vi "To Serial Form.vi"(6 "Serial Version":T1, 10 "Serializer in":refnum<class "Serializer.lvclass">, 11 "CRDS Cell Data in":refnum<class "CRDS Cell Data.lvclass">) -> (0 "error out":errorcluster, 2 "Serializer out":refnum<class "Serializer.lvclass">, 3 "CRDS Cell Data out":refnum<class "CRDS Cell Data.lvclass">)   [LabVIEW 2014, in "CRDS Cell Data.lvclass"]
uses:
  CRDS Cell Data.lvclass
  <vilib>/NI/AQ Character Lineator/Serializer/Serializer.lvclass
  <vilib>/NI/AQ Character Lineator/Serialization Common/Serial Version.ctl
  CRDS Cell Data.lvclass/CRDS Cell Data.ctl
  <vilib>/NI/AQ Character Lineator/Serializable/Insert Single.vi
  <vilib>/NI/AQ Character Lineator/Serializable/Insert Int16 Array.vi
  <vilib>/NI/AQ Character Lineator/Serializable/Insert Single Array.vi
  <vilib>/NI/AQ Character Lineator/Serializer/Insert Single.vi
  <vilib>/NI/AQ Character Lineator/Serializer/Insert Int16 Array.vi
  <vilib>/NI/AQ Character Lineator/Serializer/Insert Single Array.vi
  <vilib>/NI/AQ Character Lineator/Serializer/Read Include Default Values.vi
  Data/Data.lvclass
  <vilib>/NI/AQ Character Lineator/Serializable/Serializable.lvclass
  <vilib>/NI/AQ Character Lineator/Serialization Common/Serialization Common.lvlib
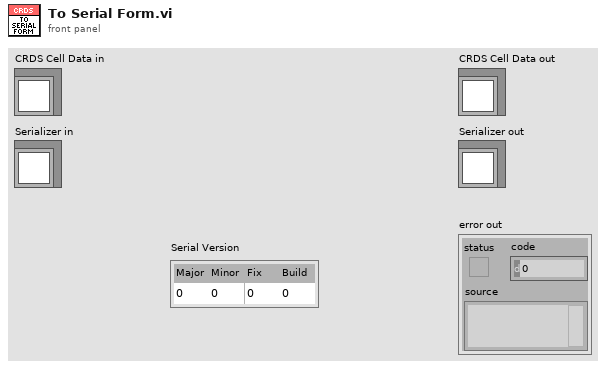
[diagram p1: front panel]
types:
  T1 = typedef "Serialization Common.lvlib/Serial Version.ctl" = cluster{"Major":u16, "Minor":u16, "Fix":u16, "Build":u16}
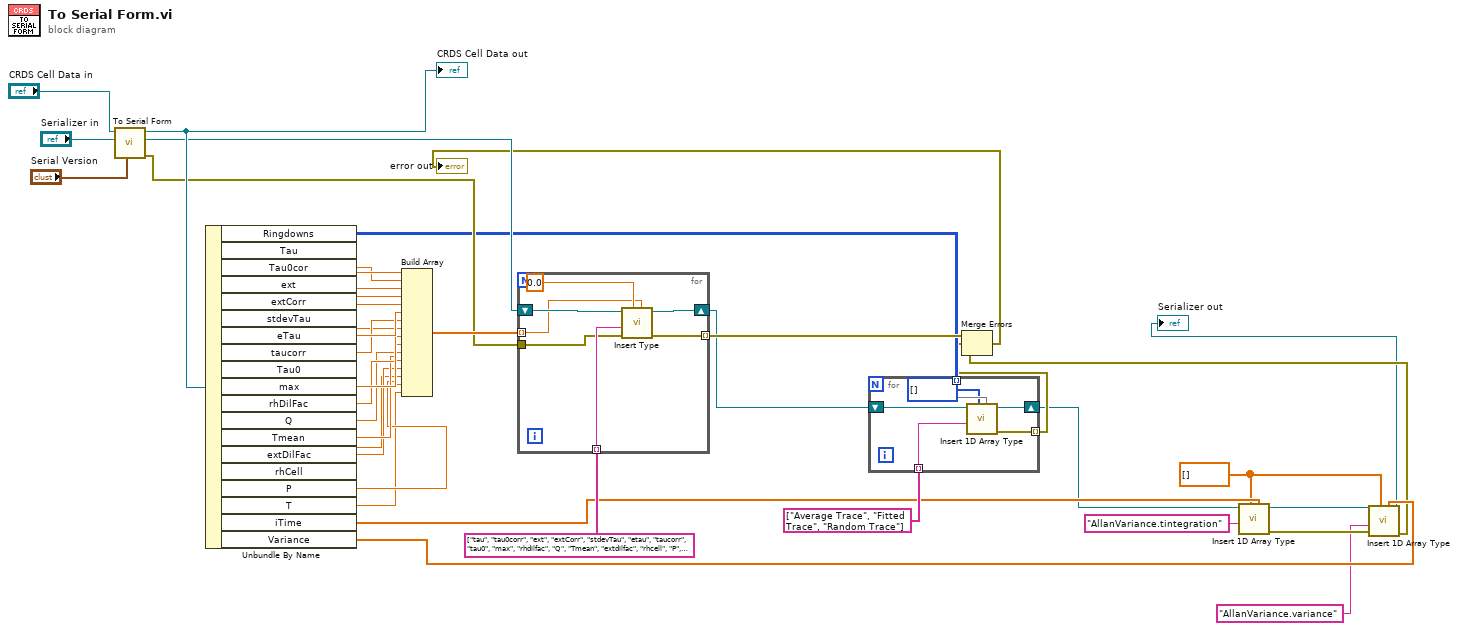
[diagram p0: block diagram]
diagram:
  w5 = sgl[] [] ("Default Value")
  n1 = call-parent "To Serial Form.vi"("Serial Version"="Serial Version", "Serializer in"="Serializer in", "Data in"="CRDS Cell Data in") -> ("error out"=w17:errorcluster, "Serializer out"=w20:refnum<class "Serializer.lvclass">, "Data out"=w37:refnum<class "CRDS Cell Data.lvclass">)  [unwired: 6 in]
  "CRDS Cell Data out" <- w37
  n2 = Unbundle By Name(w37) -> ("Ringdowns"=w14:i16[][], "Tau"=w36:sgl, "Tau0cor"=w35:sgl, "ext"=w34:sgl, "extCorr"=w33:sgl, "stdevTau"=w32:sgl, "eTau"=w31:sgl, "taucorr"=w30:sgl, "Tau0"=w29:sgl, "max"=w28:sgl, "rhDilFac"=w27:sgl, "Q"=w26:sgl, "Tmean"=w25:sgl, "extDilFac"=w24:sgl, "rhCell"=w23:sgl, "P"=w22:sgl, "T"=w21:sgl, "iTime"=w10:sgl[], "Variance"=w6:sgl[])
  n3 = Build Array(w36, w35, w34, w33, w32, w31, w30, w29, w28, w27, w26, w25, w24, w23, w22, w21) -> (w19:sgl[])
  n4 = for {
    shift-right: [w46] -> w13
    shift-left: w20 -> [w47]
    tunnel: w19 -> [w44] mode=indexing
    tunnel: string[] ["tau", "tau0corr", "ext", "extCorr", "stdevTau", "etau", "taucorr", "tau0", "max", "rhdilfac", "Q", "Tmean", "extdilfac", "rhcell", "P", "T"] -> [w43] mode=indexing
    tunnel: w17 -> [w42]
    tunnel: [w41] -> w16 mode=indexing
    n5 = call-poly <vilib>:"Insert Type.vi"("Double"=w44, "Default Value"=sgl 0.0, "error in (no error)"=w42, "Name"=w43, "Serializer in"=w47) -> ("error out"=w41:errorcluster, "Serializer out"=w46:refnum<class "Serializer.lvclass">)  [unwired: 5 in]
  }
  n6 = for {
    tunnel: w14 -> [w53] mode=indexing
    shift-right: [w50] -> w9
    shift-left: w13 -> [w51]
    tunnel: string[] ["Average Trace", "Fitted Trace", "Random Trace"] -> [w49] mode=indexing
    tunnel: [w48] -> w11 mode=indexing
    n7 = call-poly <vilib>:"Insert 1D Array Type.vi"("Integers"=w53, "Default Value"=i16[] [], "Name"=w49, "Serializer in"=w51) -> ("error out"=w48:errorcluster, "Serializer out"=w50:refnum<class "Serializer.lvclass">)  [unwired: 6 in]
  }
  n8 = call-poly <vilib>:"Insert 1D Array Type.vi"("Singles"=w10, "Default Value"=w5, "Name"="AllanVariance.tintegration", "Serializer in"=w9) -> ("error out"=w4:errorcluster, "Serializer out"=w7:refnum<class "Serializer.lvclass">)  [unwired: 6 in]
  n9 = call-poly <vilib>:"Insert 1D Array Type.vi"("Singles"=w6, "Default Value"=w5, "error in (no error)"=w4, "Name"="AllanVariance.variance", "Serializer in"=w7) -> ("error out"=w3:errorcluster, "Serializer out"=→"Serializer out":refnum<class "Serializer.lvclass">)  [unwired: 5 in]
  n10 = Merge Errors(w16, w11, w3) -> (→"error out":errorcluster)
